vi "TempControlWithBool.vi"(6 "error in":errorcluster, 9 "INPUT":string) -> (0 "error out":errorcluster, 2 "out":dbl, 4 "Valid(t)":bool)   [LabVIEW 2018]
doc: "Input a String and return a Number.\n\nLeave String blank, and a number returns."
panel:
  # "Input a number get a valid T\nInput a keyword: room, ambient, or skip, or empty returns false"
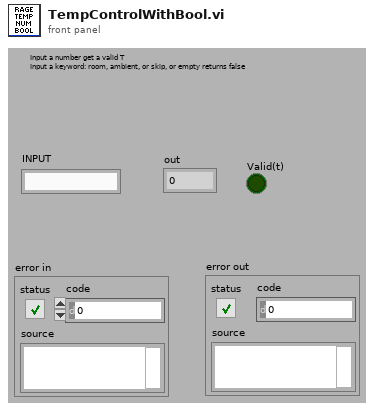
[diagram p1: front panel]
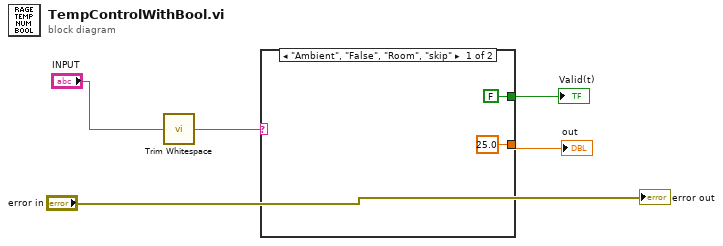
[diagram p0: block diagram]
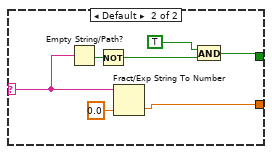
[diagram p2: hidden frame]
diagram:
  n1 = call <vilib>:"Trim Whitespace.vi"("string"="INPUT") -> ("trimmed string"=w1:string)  [unwired: 1 in]
  n2 = case shown="\"Ambient\", \"False\", \"Room\", \"skip\"" w1 {
    selector: w1 -> [_ w12]
    tunnel: [25.0 w13] -> w5
    tunnel: [FALSE w8] -> w4
    frame "Ambient", "False", "Room", "skip" {
    }
    frame Default {
      n3 = Empty String/Path?(string/path=w12) -> (empty?=w11:bool)
      n4 = Not(x=w11) -> (.not. x?=w10:bool)
      n5 = Fract/Exp String To Number(string=w12, default (0 dbl)=0.0 ("default (0 DBL)")) -> (number=w13:dbl)  [unwired: 2 in, 1 out]
      n6 = And(x=TRUE, y=w10) -> (x .and. y?=w8:bool)
    }
  }
  "out" <- w5
  "Valid(t)" <- w4
  "error out" <- "error in"
